vi "ChangeAIParametersCauseStrikers.vi"(7 "AI Parameters":T1={"GotoKick"={"Dist do cone a frente"=150.0, "attacker farback"=1500.0, "Perto"=300.0, "min dist to kick"=150.0, "kick eps"=0.0, "Time to transition"=0.05}, "Attacker"={"CC chute"=0.09, "CC passe"=0.045, "Kick Force"=100.0, "ball-robot Kick"=200.0, "ball-robot Pass"=0.3, "drible\nAttk"=FALSE}, "Defender"={"D max"=1700.0, "Vel p/ robô av"=1000.0, "Kick Force"=100.0, "D atk-def"=0.0, "D farback"=0.0, "drible\ndef"=FALSE, "drible\ngoalie"=FALSE}, "Timeout"={"Field/v in x"=6.0, "Dist Robots"=300, "Dist up in y"=300}, "Pose Striker"={"dist"=200.0, "Numeric"=-4.0, "dist 2"=200.0, "drible\nstriker"=FALSE}, "Dist Stop"=300.0, "D ball out"=200, "D central gap "=150.0, "T pass"=0.0, "Force ++"=0.0, "range kick"=0.0, "Chute alto"=TRUE, "Marcador novo"=TRUE, "drible"=FALSE, "D drible"=300.0, "Versão Striker"=enum."3", "Defesa"=enum."ManMark", "Marcador"=enum."Marcar Segndo mais perigoso", "Receptor passe"=enum."2nd Striker"} {"D drible" format="%#_13g"; "D central gap" format="%#_13g"; "Dist Stop" format="%#_13g"; "Pose Striker"."Numeric" format="%#_13g"; "Defender"."Kick Force" format="%#_13g"; "Defender"."Vel p/ robô av" format="%#_13g"; "Attacker"."ball-robot Kick" format="%#_13g"; "Attacker"."Kick Force" format="%#_13g"; "Attacker"."CC passe" format="%#_13g"; "Attacker"."CC chute" format="%#_13g"; "GotoKick"."kick eps" format="%#_13g"; "GotoKick"."min dist to kick" format="%#_13g"; "GotoKick"."Perto" format="%#_13g"; "GotoKick"."attacker farback" format="%#_13g"; "GotoKick"."Dist do cone a frente" format="%#_13g"}, 11 "IA State Input":T2={"our_robots"=[], "enemy_robots"=[], "balls"=[], "geometry"={"line_width"=0, "field_length"=0, "field_width"=0, "boundary_width"=0, "referee_width"=0, "goal_width"=0, "goal_depth"=0, "goal_wall_width"=0, "center_circle_radius"=0, "defense_radius"=0, "defense_stretch"=0, "free_kick_from_defense_dist"=0, "penalty_spot_from_field_line_dist"=0, "penalty_line_from_spot_dist"=0}, "IA Judge"={"stage"="", "command"="", "our_goalie_id"=0.0, "enemy_goalie_id"=0.0, "command enum"=enum."Halt", "Time"=enum."Azul"}, "Received Timestamp"=timestamp(0 s since 1904-01-01), "Events"={"Touch"=FALSE, "Ball out"=FALSE, "id touch"=0.0, "Ball out of \nVision"=FALSE, "Ball inside \nGoalie area"=FALSE, "Robot not responding"=FALSE, "Robots responding status"=[1.0, 1.0, 1.0, 1.0, 1.0, 1.0], "Enemy Ball \nPossession"=FALSE, "Pass State"=FALSE, "id end of pass"=0.0, "Kick"=FALSE, "Id ini Possession"=0.0, "Ball Possesion"=FALSE, "Id Possesion"=0.0, "Direct Kick"=FALSE, "2nd Strk Ativo"=FALSE}}) -> (6 "AI Parameters Output":T1={"GotoKick"={"Dist do cone a frente"=150.0, "attacker farback"=1500.0, "Perto"=300.0, "min dist to kick"=150.0, "kick eps"=0.0, "Time to transition"=0.05}, "Attacker"={"CC chute"=0.09, "CC passe"=0.045, "Kick Force"=100.0, "ball-robot Kick"=200.0, "ball-robot Pass"=0.3, "drible\nAttk"=FALSE}, "Defender"={"D max"=1700.0, "Vel p/ robô av"=1000.0, "Kick Force"=100.0, "D atk-def"=0.0, "D farback"=0.0, "drible\ndef"=FALSE, "drible\ngoalie"=FALSE}, "Timeout"={"Field/v in x"=6.0, "Dist Robots"=300, "Dist up in y"=300}, "Pose Striker"={"dist"=200.0, "Numeric"=-4.0, "dist 2"=200.0, "drible\nstriker"=FALSE}, "Dist Stop"=300.0, "D ball out"=200, "D central gap "=150.0, "T pass"=0.0, "Force ++"=0.0, "range kick"=0.0, "Chute alto"=TRUE, "Marcador novo"=TRUE, "drible"=FALSE, "D drible"=300.0, "Versão Striker"=enum."3", "Defesa"=enum."ManMark", "Marcador"=enum."Marcar Segndo mais perigoso", "Receptor passe"=enum."2nd Striker"} {"D drible" format="%#_13g"; "D central gap" format="%#_13g"; "Dist Stop" format="%#_13g"; "Pose Striker"."Numeric" format="%#_13g"; "Defender"."Kick Force" format="%#_13g"; "Defender"."Vel p/ robô av" format="%#_13g"; "Attacker"."ball-robot Kick" format="%#_13g"; "Attacker"."Kick Force" format="%#_13g"; "Attacker"."CC passe" format="%#_13g"; "Attacker"."CC chute" format="%#_13g"; "GotoKick"."kick eps" format="%#_13g"; "GotoKick"."min dist to kick" format="%#_13g"; "GotoKick"."Perto" format="%#_13g"; "GotoKick"."attacker farback" format="%#_13g"; "GotoKick"."Dist do cone a frente" format="%#_13g"})   [LabVIEW 2017]
uses:
  AI Parameters.ctl
  Core/AI Input.ctl
  Core/AI Robot.ctl
  Functions Enum.ctl
  AttackerStates.ctl
  Path Planning/RRT/PathDests.ctl
  Path Planning/RRT/PathDest.ctl
  Core/AI Ball.ctl
  Core/Field Size.ctl
  Core/AI Judge.ctl
  Command Enum.ctl
  Util/Events/Events.ctl
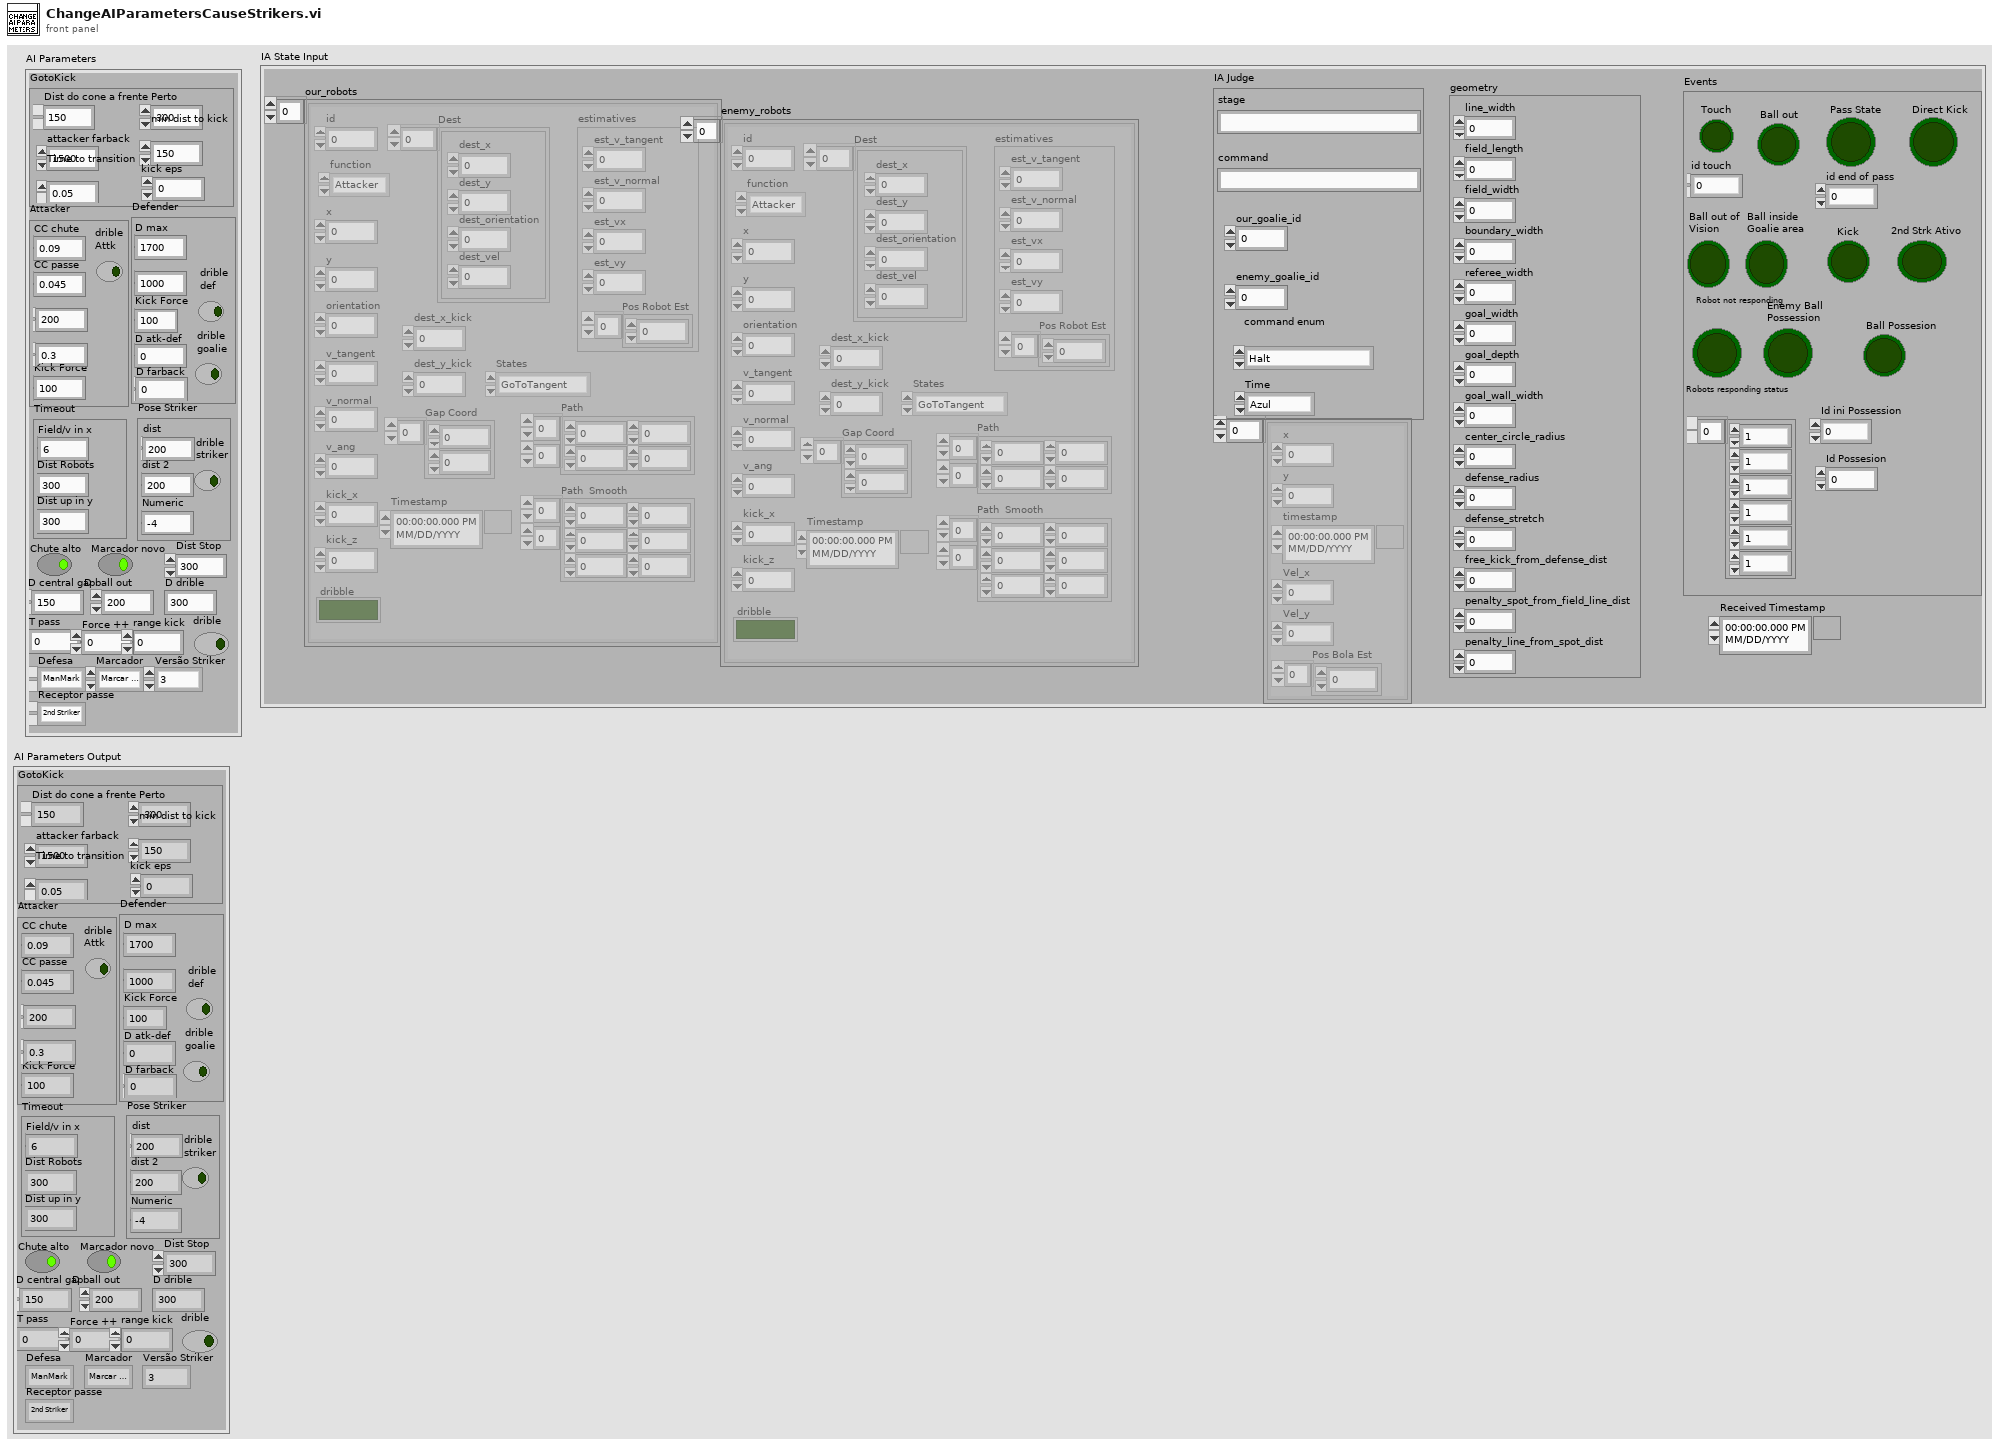
[diagram p1: front panel]
types:
  T1 = typedef "AI Parameters.ctl" = cluster{"GotoKick":cluster{"Dist do cone a frente":dbl, "attacker farback":dbl, "Perto":dbl, "min dist to kick":dbl, "kick eps":dbl, "Time to transition":dbl}, "Attacker":cluster{"CC chute":dbl, "CC passe":dbl, "Kick Force":dbl, "ball-robot Kick":dbl, "ball-robot Pass":dbl, "drible\nAttk":bool}, "Defender":cluster{"D max":dbl, "Vel p/ robô av":dbl, "Kick Force":dbl, "D atk-def":dbl, "D farback":dbl, "drible\ndef":bool, "drible\ngoalie":bool}, "Timeout":cluster{"Field/v in x":dbl, "Dist Robots":u32, "Dist up in y":u32}, "Pose Striker":cluster{"dist":dbl, "Numeric":dbl, "dist 2":dbl, "drible\nstriker":bool}, "Dist Stop":dbl, "D ball out":i32, "D central gap ":dbl, "T pass":dbl, "Force ++":dbl, "range kick":dbl, "Chute alto":bool, "Marcador novo":bool, "drible":bool, "D drible":dbl, "Versão Striker":enum16{"Auto", "3", "2", "1"}, "Defesa":enum16{"ManMark", "Barreira"}, "Marcador":enum16{"Marcar Segndo mais perigoso", "Marcar o mais perigoso"}, "Receptor passe":enum16{"Auto", "2nd Striker", "Striker"}}
  T2 = typedef "AI Input.ctl" = cluster{"our_robots":T3[], "enemy_robots":T3[], "balls":T8[], "geometry":T9, "IA Judge":T10, "Received Timestamp":timestamp, "Events":T12}
  T3 = typedef "AI Robot.ctl" = cluster{"id":u32, "function":T4, "x":dbl, "y":dbl, "orientation":dbl, "v_tangent":dbl, "v_normal":dbl, "v_ang":dbl, "kick_x":dbl, "kick_z":dbl, "dribble":bool, "Timestamp":timestamp, "estimatives":cluster{"est_v_tangent":dbl, "est_v_normal":dbl, "est_vx":dbl, "est_vy":dbl, "Pos Robot Est":dbl[]}, "dest_x_kick":dbl, "dest_y_kick":dbl, "Gap Coord":dbl[], "States":T5, "Path ":dbl[][], "Path  Smooth":dbl[][], "Dest":T6}
  T4 = typedef "Functions Enum.ctl" = enum16{"2nd Striker", "Attacker", "Goalie", "Defender", "Striker", "Goto 0", "Dummy", "Kicker", "ZigZag 0", "ZigZag 1", "ZigZag 2", "ZigZag 3", "ZigZag 4", "ZigZag 5", "ZigZag 6", "ZigZag 7", "ZigZag 8", ""}
  T5 = typedef "AttackerStates.ctl" = enum16{"Pass", "GoToTangent", "BallGetting", "GoToKick", ""}
  T6 = typedef "PathDests.ctl" = T7[]
  T7 = typedef "PathDest.ctl" = cluster{"dest_x":dbl, "dest_y":dbl, "dest_orientation":dbl, "dest_vel":dbl}
  T8 = typedef "AI Ball.ctl" = cluster{"x":dbl, "y":dbl, "timestamp":timestamp, "Vel_x":dbl, "Vel_y":dbl, "Pos Bola Est":dbl[]}
  T9 = typedef "Field Size.ctl" = cluster{"line_width":u32, "field_length":u32, "field_width":u32, "boundary_width":u32, "referee_width":u32, "goal_width":u32, "goal_depth":u32, "goal_wall_width":u32, "center_circle_radius":u32, "defense_radius":u32, "defense_stretch":u32, "free_kick_from_defense_dist":u32, "penalty_spot_from_field_line_dist":u32, "penalty_line_from_spot_dist":u32}
  T10 = typedef "AI Judge.ctl" = cluster{"stage":string, "command":string, "our_goalie_id":dbl, "enemy_goalie_id":dbl, "command enum":T11, "Time":enum16{"Azul", "Amarelo"}}
  T11 = typedef "Command Enum.ctl" = enum16{"Halt", "Stop", "Force Start", "PKA Normal Start", "Prepare Kickoff Ally", "PKE Normal Start", "Prepare Kickoff Enemy", "Prepare Penalty Ally", "PPA Normal Start", "Prepare Penalty Enemy", "PPE Normal Start", "Direct Free Enemy", "Direct Free Ally", "Indirect Free Enemy", "Indirect Free Ally", "Timeout Enemy", "Timeout Ally", "Goal Enemy", "Goal Ally", "Ball Placement Enemy", "Ball Placement Ally", "Normal Half Time", "Extra Time Break", "Extra Half Time", "None", "Post Game"}
  T12 = typedef "Events.ctl" = cluster{"Touch":bool, "Ball out":bool, "id touch":dbl, "Ball out of \nVision":bool, "Ball inside \nGoalie area":bool, "Robot not responding":bool, "Robots responding status":dbl[], "Enemy Ball \nPossession":bool, "Pass State":bool, "id end of pass":dbl, "Kick":bool, "Id ini Possession":dbl, "Ball Possesion":bool, "Id Possesion":dbl, "Direct Kick":bool, "2nd Strk Ativo":bool}
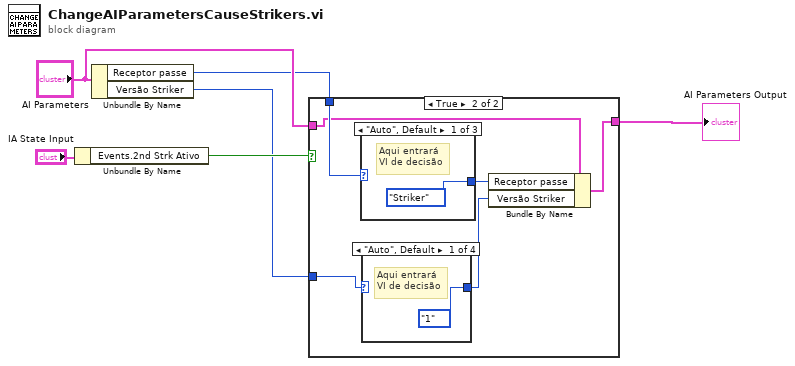
[diagram p0: block diagram]
diagram:
  n1 = Unbundle By Name("IA State Input") -> ("Events.2nd Strk Ativo"=w5:bool)
  n2 = Unbundle By Name("AI Parameters") -> ("Receptor passe"=w2:enum16{"Auto", "2nd Striker", "Striker"}, "Versão Striker"=w1:enum16{"Auto", "3", "2", "1"})
  n3 = case shown="True" w5 {
    tunnel: [w7 w11] -> w4
    tunnel: "AI Parameters" -> [w7 w12]
    tunnel: w2 -> [_ w13]
    tunnel: w1 -> [_ w9]
    frame False {
    }
    frame True {
      n4 = case shown="\"Auto\", Default" w13 {
        selector: w13 -> [_ w19 w20]
        tunnel: [enum16{"Auto", "2nd Striker", "Striker"}."Striker" ("Receptor passe") w19 w20] -> w10
        frame "Auto", Default {
          # "Aqui entrará\nVI de decisão"
        }
        frame "Striker" {
        }
        frame "2nd Striker" {
        }
      }
      n5 = case shown="\"Auto\", Default" w9 {
        selector: w9 -> [_ w15 w16 w17]
        tunnel: [enum16{"Auto", "3", "2", "1"}."1" ("Versão Striker") w15 w16 w17] -> w8
        frame "Auto", Default {
          # "Aqui entrará\nVI de decisão"
        }
        frame "1" {
        }
        frame "2" {
        }
        frame "3" {
        }
      }
      n6 = Bundle By Name(cluster=w12, "Receptor passe"=w10, "Versão Striker"=w8) -> (w11:T1)
    }
  }
  "AI Parameters Output" <- w4
